vi "Transient Memory.vi"   [LabVIEW 2018, in "TDK-Lambda Z.lvlib"]
uses:
  TDK-Lambda Z.lvlib
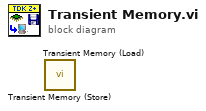
[diagram p0: block diagram]
diagram:
  n1 = call "Transient Memory (Store).vi"() -> ()  [unwired: 10 in, 2 out]
  n2 = call "Transient Memory (Load).vi"() -> ()  [unwired: 10 in, 2 out]
